vi "Get All LogMeasData from Q.vi"(8 "error in (no error)":errorcluster) -> (0 "error out":errorcluster, 1 "MeasData[] out":T1[](array[typedef]), 2 "NumElements":i32, 3 "orData out":T2)   [LabVIEW 2017]
doc: "Developed by Kevin Thompson\nThompson Engineering, LLC\nkevin@thompsonengineering.net"
uses:
  TD MeasData QRef.ctl
  TD MeasData--cluster.ctl
  GBL DataQ Ref.vi
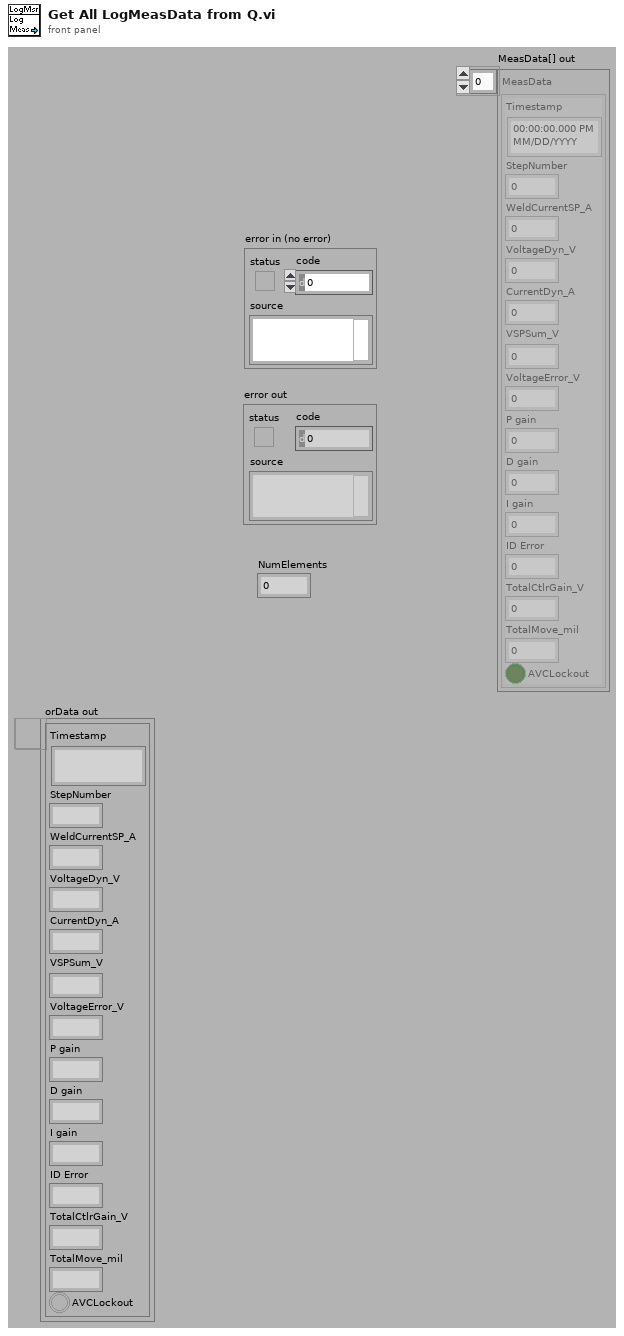
[diagram p1: front panel]
types:
  T1 = typedef "TD MeasData--cluster.ctl" = cluster{"Timestamp":timestamp, "StepNumber":i32, "WeldCurrentSP_A":dbl, "VoltageDyn_V":dbl, "CurrentDyn_A":dbl, "VSPSum_V":dbl, "VoltageError_V":dbl, "P gain":dbl, "D gain":dbl, "I gain":dbl, "ID Error":dbl, "TotalCtlrGain_V":dbl, "TotalMove_mil":dbl, "AVCLockout":bool}
  T2 = typedef "TD MeasData QRef.ctl" = refnum<queue>
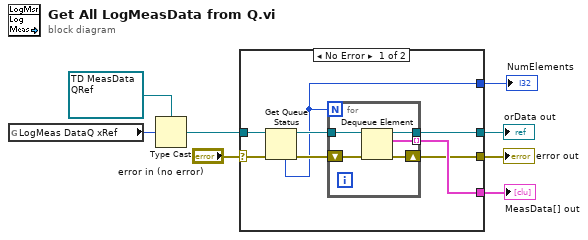
[diagram p0: block diagram]
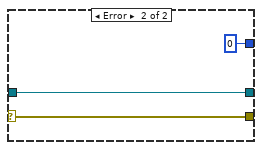
[diagram p2: hidden frame]
diagram:
  n1 = global read "GBL DataQ Ref.vi" "LogMeas DataQ xRef"() -> (w1:u32)
  n2 = Type Cast(type=T2 refnum ("orData out"), x=w1) -> (*(type *) &x=w5:T2)
  n3 = case shown="No Error" "error in (no error)" {
    selector: "error in (no error)" -> [w16 w23]
    tunnel: w5 -> [w15 w24]
    tunnel: [w10 w23] -> w8
    tunnel: [w14 w24] -> w7
    tunnel: [w11 _] -> w4
    tunnel: [w9 0 ("# elements in queue")] -> w3
    frame No Error {
      n4 = Get Queue Status(queue=w15, error in (no error)=w16) -> (queue out=w13:T2, error out=w12:errorcluster, # elements in queue=w9:i32)  [unwired: 1 in, 5 out]
      n5 = for {
        N: w9 -> [_]
        tunnel: [w21] -> w11 mode=indexing
        tunnel: [w20] -> w14
        tunnel: w13 -> [w19]
        shift-right: [w18] -> w10
        shift-left: w12 -> [w17]
        n6 = Dequeue Element(queue=w19, error in (no error)=w17) -> (queue out=w20:T2, element=w21:T1, error out=w18:errorcluster)  [unwired: 1 in, 1 out]
      }
    }
    frame Error {
    }
  }
  "orData out" <- w7
  "error out" <- w8
  "MeasData[] out" <- w4
  "NumElements" <- w3
